vi "Msg.vi"(7 "jettl in":refnum<class "jettl.lvclass">, 11 "Teardown Msg Strategy in":refnum<class "Teardown Msg Strategy.lvclass">) -> (5 "jettl out":refnum<class "jettl.lvclass">)   [LabVIEW 2021, in "jettl.lvlib" / "Teardown Msg Strategy.lvlib" / "Teardown Msg Strategy.lvclass"]
uses:
  Teardown Msg Strategy.lvclass
  Teardown Msg Strategy.lvclass/Teardown Msg Strategy.ctl
  Teardown/Teardown.lvclass
  jettl/jettl.lvclass
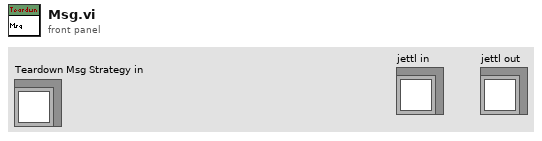
[diagram p1: front panel]
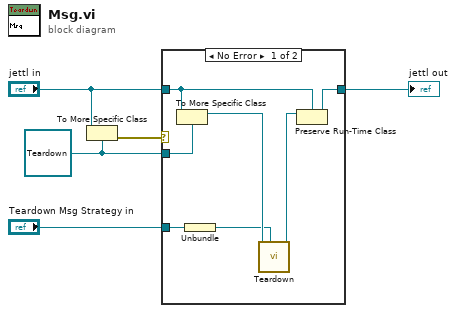
[diagram p0: block diagram]
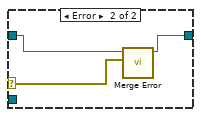
[diagram p2: hidden frame]
diagram:
  w4 = refnum<class "Teardown.lvclass"> refnum ("Destroy.lvlib:Destroy.lvclass")
  n1 = To More Specific Class(target class=w4, reference="jettl in") -> (error out=w5:errorcluster)  [unwired: 1 in, 1 out]
  n2 = case shown="No Error" w5 {
    selector: w5 -> [_ w13]
    tunnel: [w10 w14] -> w2
    tunnel: "jettl in" -> [w11 w15]
    tunnel: w4 -> [w12 _]
    tunnel: "Teardown Msg Strategy in" -> [w7 _]
    frame No Error {
      n3 = To More Specific Class(target class=w12, reference=w11) -> (specific class reference=w9:refnum<class "Teardown.lvclass">)  [unwired: 1 in, 1 out]
      n4 = Unbundle "Unbundle"(w7) -> (w6:refnum<class "Sender.lvclass">)
      n5 = call-dynamic "Teardown.vi"("Sender"=w6, "Teardown in"=w9) -> ("Teardown out"=w8:refnum<class "Teardown.lvclass">)  [unwired: 9 in]
      n6 = Preserve Run-Time Class(object in=w8, 2:w11) -> (object out=w10:refnum<class "jettl.lvclass">)  [unwired: 1 in, 1 out]
    }
    frame Error {
      n7 = call-dynamic "Merge Error.vi"("Error"=w13, "jettl in"=w15) -> ("jettl out"=w14:refnum<class "jettl.lvclass">)  [unwired: 9 in]
    }
  }
  "jettl out" <- w2
